vi "FPGA Main.vi"() -> ()   [LabVIEW 2022 SP3]
uses:
  <vilib>/rvi/Emulation/niFpgaGetClockAttributes.vi
  <vilib>/rvi/Emulation/niFpgaSctlEmulationGetInTimedLoop.vi
  <vilib>/rvi/Emulation/niFpgaEmulationReportErrorSimple.vi
  <vilib>/rvi/eio/common/nirviEmuTemplateMethod_errors.vi
  <vilib>/rvi/Emulation/niFpgaCriticalErrorInLSC.vi
  <vilib>/eio/EIONode/EIONode.xnode
panel:
  in  "Waiting Time":u32 caption="计数器(mSec)"
  out "x-y":u32
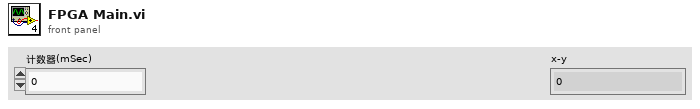
[diagram p1: front panel]
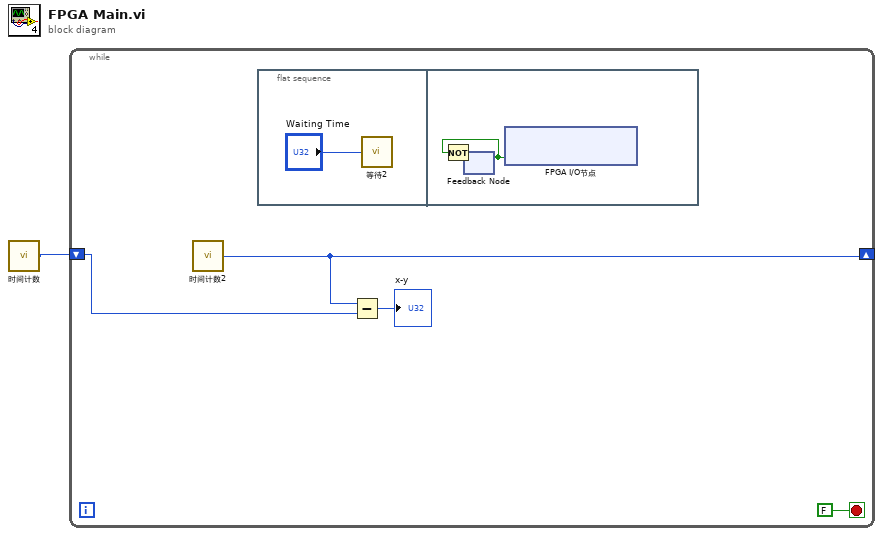
[diagram p0: block diagram]
diagram:
  n1 = call "时间计数"() -> ("Tick Count(Ticks)"=w1:u32)
  n2 = while {
    shift-right: [w5] -> _
    shift-left: w1 -> [w4]
    stop <- FALSE stop-if-true
    n3 = call "时间计数2"() -> ("Tick Count(Ticks)"=w5:u32)
    n4 = flat-sequence {
      frame #0 {
        n5 = call "等待2"("Count(mSec)"="Waiting Time") -> ()  [unwired: 1 out]
      }
      frame #1 {
        n6 = feedback #1() -> (w7:bool)  [unwired: 1 in]
        n7 = Not(x=w7) -> (.not. x?=w8:bool)
        n8 = feedback-in #1(w8) -> ()
        n9 = xnode "FPGA I/O节点"("模块7/User LED"=w7) -> ()  [unwired: 1 in, 1 out]
      }
    }
    n10 = Subtract(x=w5, y=w4) -> (x-y=→"x-y":u32)
  }
